vi "EX_NOR.vi"() -> ()   [LabVIEW 2024]
panel:
  out "x .or. y?":bool
  in  "y":bool
  in  "x":bool
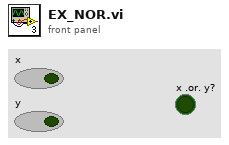
[diagram p1: front panel]
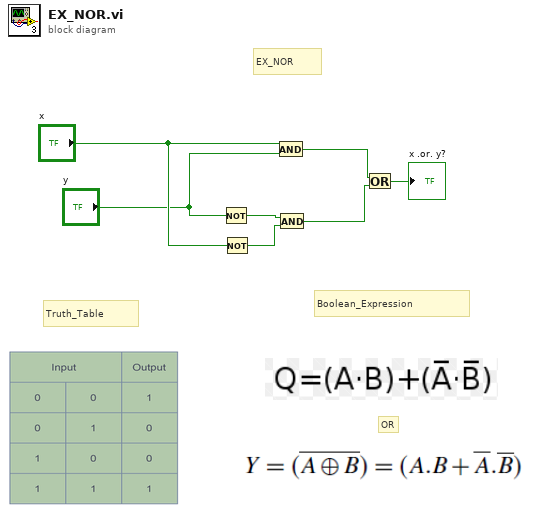
[diagram p0: block diagram]
diagram:
  # "EX_NOR"
  # "Boolean_Expression"
  # "Truth_Table"
  # "OR"
  n1 = Not(x="y") -> (.not. x?=w4:bool)
  n2 = Not(x="x") -> (.not. x?=w5:bool)
  n3 = And(x="x", y="y") -> (x .and. y?=w7:bool)
  n4 = And(x=w4, y=w5) -> (x .and. y?=w6:bool)
  n5 = Or(x=w7, y=w6) -> (x .or. y?=→"x .or. y?":bool)
